vi "connection.list.vi"(8 "error in":errorcluster, 9 "Include Archived?":bool, 10 "Workspace RIDs (all)":string[](array[string]), 11 "Nominal Client in":refnum<class "Nominal Client.lvclass">) -> (0 "error out":errorcluster, 1 "Response":string, 2 "Connections":T1(array[cluster]), 3 "Nominal Client out":refnum<class "Nominal Client.lvclass">)   [LabVIEW 2020, in "Nominal Client.lvclass"]
doc: "Lists all connections"
uses:
  Nominal Client.lvclass
  28804fc9-aee6-4b6e-ba11-1ba961eefadd.vi
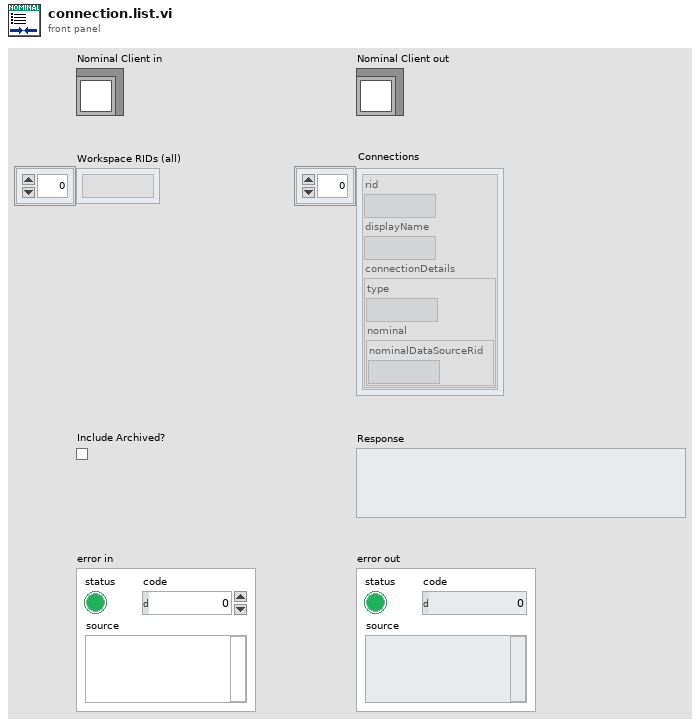
[diagram p1: front panel]
types:
  T1 = cluster{"rid":string, "displayName":string, "connectionDetails":cluster{"type":string, "nominal":cluster{"nominalDataSourceRid":string}}}[]
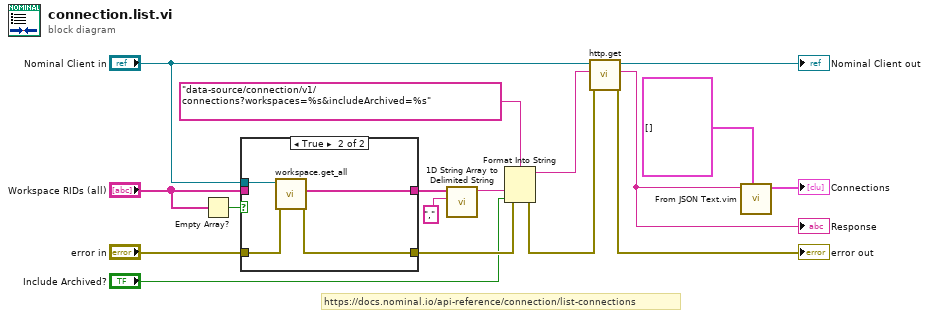
[diagram p0: block diagram]
diagram:
  # "https://docs.nominal.io/api-reference/connection/list-connections"
  n1 = Empty Array?(array="Workspace RIDs (all)") -> (empty?=w11:bool)
  n2 = case shown="True" w11 {
    tunnel: "Nominal Client in" -> [_ w23]
    tunnel: "Workspace RIDs (all)" -> [w19 _]
    tunnel: [w19 w20] -> w9
    tunnel: "error in" -> [w18 w22]
    tunnel: [w18 w21] -> w4
    frame False {
    }
    frame True {
      n3 = call "workspace.get_all.vi"("error in"=w22, "Nominal Client in"=w23) -> ("error out"=w21:errorcluster, "Workspace RIDs"=w20:string[])  [unwired: 5 in, 3 out]
    }
  }
  n4 = call <vilib>:"1D String Array to Delimited String.vi"("delimiter"=",", "string array"=w9) -> ("delimited string"=w6:string)  [unwired: 9 in]
  n5 = Format Into String(format string="data-source/connection/v1/connections?workspaces=%s&includeArchived=%s" ("Path"), error in=w4, w6, "Include Archived?") -> (resulting string=w5:string, error out=w2:errorcluster)  [unwired: 1 in]
  n6 = call "http.get.vi"("error in"=w2, "Path"=w5, "Nominal Client in"="Nominal Client in") -> ("error out"=→"error out":errorcluster, "Response"=w15:string, "Nominal Client out"=→"Nominal Client out":refnum<class "Nominal Client.lvclass">)  [unwired: 5 in, 1 out]
  "Response" <- w15
  n7 = call "From JSON Text.vim"("Data Type and Default Value"=T1 [] ("Connections"), "JSON"=w15) -> ("Data out"=→"Connections":T1)  [unwired: 8 in, 1 out]
